vi "Eth Status Read Stop_com.vi"(7 "Status Reference":T1, 8 "error in (no error)":errorcluster) -> (0 "error out":errorcluster, 1 "Stop":bool)   [LabVIEW 2019, in "Eth Status.lvlib"]
uses:
  Eth Status.lvlib
  Ctl/Status.ctl
  MB_TCP2/MB_TCP_State.ctl
  MB_TCP2/MB_TCP.lvclass
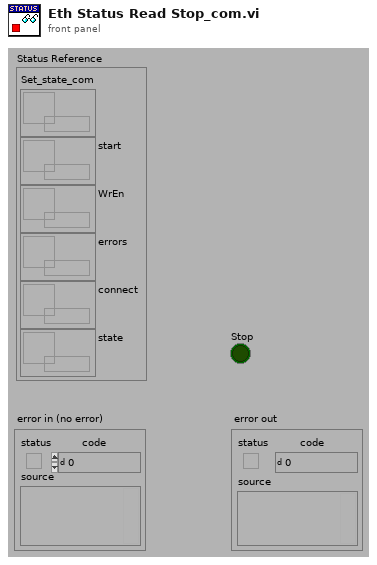
[diagram p1: front panel]
types:
  T1 = typedef "Eth Status.lvlib/Status.ctl" = cluster{"Set_state_com":refnum<data-value>, "start":refnum<data-value>, "WrEn":refnum<data-value>, "errors":refnum<data-value>, "connect":refnum<data-value>, "state":refnum<data-value>}
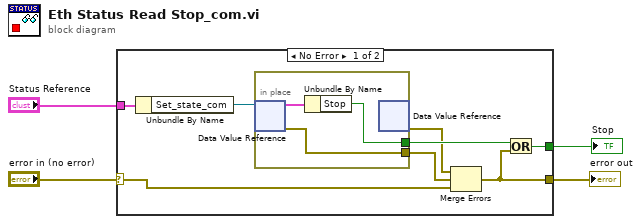
[diagram p0: block diagram]
diagram:
  n1 = case shown="No Error" "error in (no error)" {
    selector: "error in (no error)" -> [w6 w16]
    tunnel: [w5 w16] -> w4
    tunnel: "Status Reference" -> [w12 _]
    tunnel: [w7 _] -> w2
    frame No Error {
      n2 = Unbundle By Name(w12) -> ("Set_state_com"=w11:refnum<data-value>)
      n3 = in-place {
        in-place-border: [w13] -> w10
        in-place-border: [w15] -> w8
        n4 = in-place-dvr #1(w11) -> (w14:cluster{"Start":bool, "WrEn":bool, "Stop":bool}, w15:errorcluster)
        n5 = Unbundle By Name(w14) -> ("Stop"=w13:bool)
        n6 = in-place-dvr #1() -> (w9:errorcluster)  [unwired: 1 in, 1 out]
      }
      n7 = Merge Errors(w9, w8, w6) -> (w5:errorcluster)
      n8 = Or(x=w10, y=w5) -> (x .or. y?=w7:bool)
    }
    frame Error {
    }
  }
  "error out" <- w4
  "Stop" <- w2
